vi "Undersample_HT.vi"(6 "error in (no error)":errorcluster, 7 "Unit Info":string="Unit1", 8 "U/S Frequency":i32=2400, 9 "U/S Location":string(combo)="VCO") -> (0 "error out":errorcluster, 2 "Cycle-Cycle Jitter":string, 3 "Total RMS Jitter":string)   [LabVIEW 2011]
doc: "This VI undersamples a selected signal from the HT Link 0 PLL at a specified frequency.\n\nInputs:\n1. U/S Location: Part of PLL loop to be undersamles (VCO, PllOut, VCO_Z, Spine, etc).\n2. U/S Frequency: Frequency at which the PLL to be undersampled is running (2400, 2600, etc.)\n3. Unit Info: Information about the unit to attach to undersampling results file.\n\nOutputs:\n1. Total RMS Jitter: The total RMS Jitter as read from the resultspectrum file.\n2. Cycle-Cycle Jitter: The Cycle-Cycle Jitter as read from the result spectrum file."
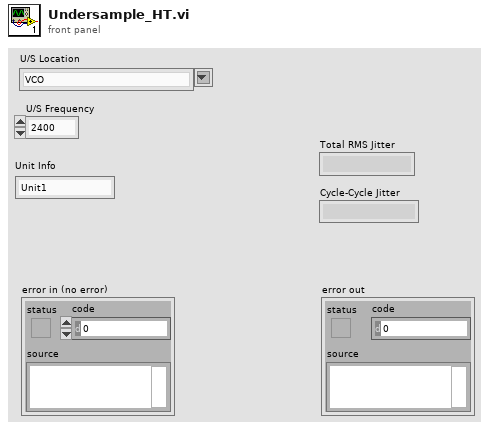
[diagram p1: front panel]
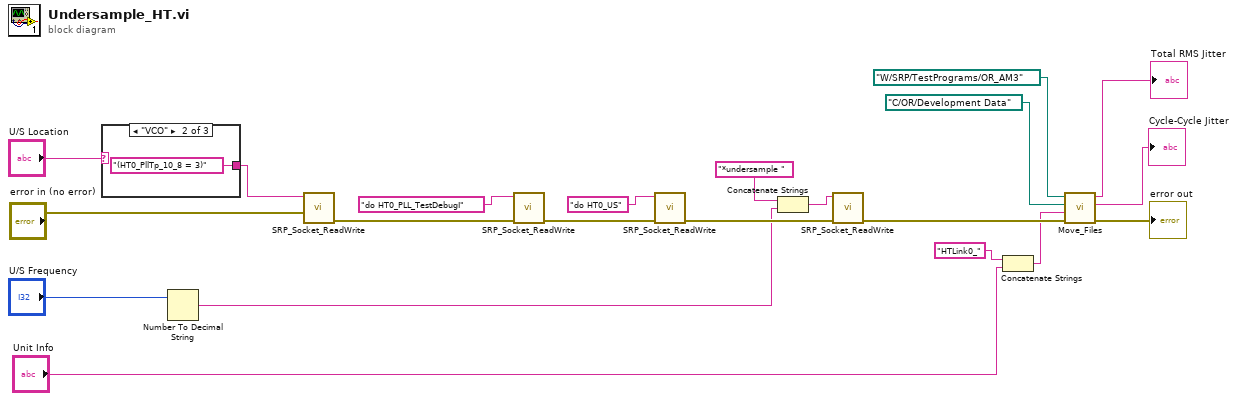
[diagram p0: block diagram]
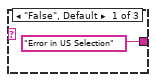
[diagram p2: hidden frame]
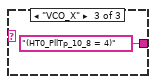
[diagram p3: hidden frame]
diagram:
  n1 = case shown="\"VCO\"" "U/S Location" {
    tunnel: ["Error in US Selection" "(HT0_PllTp_10_8 = 3)" "(HT0_PllTp_10_8 = 4)"] -> w6
    frame "False", Default {
    }
    frame "VCO" {
    }
    frame "VCO_X" {
    }
  }
  n2 = Number To Decimal String(number="U/S Frequency") -> (decimal integer string=w1:string)  [unwired: 1 in]
  n3 = call "SRP_Socket_ReadWrite.vi"("error in (no error)"="error in (no error)", "Data In"=w6) -> ("error out"=w16:errorcluster)  [unwired: 7 in, 1 out]
  n4 = call "SRP_Socket_ReadWrite.vi"("error in (no error)"=w16, "Data In"="do HT0_PLL_TestDebugI") -> ("error out"=w18:errorcluster)  [unwired: 7 in, 1 out]
  n5 = call "SRP_Socket_ReadWrite.vi"("error in (no error)"=w18, "Data In"="do HT0_US") -> ("error out"=w15:errorcluster)  [unwired: 7 in, 1 out]
  n6 = Concatenate Strings("*undersample ", w1) -> (w7:string)
  n7 = call "SRP_Socket_ReadWrite.vi"("error in (no error)"=w15, "Data In"=w7) -> ("error out"=w13:errorcluster)  [unwired: 7 in, 1 out]
  n8 = Concatenate Strings("HTLink0_" ("string"), "Unit Info") -> (w10:string)
  n9 = call "Move_Files.vi"("error in"=w13, "Unit Information"=w10, "Target Directory to Save U/S Files"=path "C:/OR/Development Data", "Location of U/S Files"=path "W:/SRP/TestPrograms/OR_AM3") -> ("error out"=→"error out":errorcluster, "Cycle-Cycle-Jitter"=→"Cycle-Cycle Jitter":string, "Total RMS Jitter"=→"Total RMS Jitter":string)  [unwired: 5 in]
